vi "Write Config to File.vi"() -> ()   [LabVIEW 2014]
uses:
  General/Controls/System Parameters.ctl
  Hardware/Table Stage/Controls/Translation Stage Cluster.ctl
  General/Controls/Translation Stage Types.ctl
  <vilib>/Utility/config.llb/NI_LVConfig.lvlib
panel:
  in  "System Parameters":T1={"OCT"={"Focal Length"=0.0}, "Vibratome"={"Z Bottom"=0.0, "Pre Cut Dwell"=0.0, "Blade Frequency"=0.0, "Slice Speed"=0.0, "Post Cut Dwell"=0.0, "Ramp Time"=0.0, "Start X"=0.0, "Start Y"=0.0}, "Table Stages"={"X Stage"={"Position"=0.0, "Is.Enabled?"=FALSE, "Is.Connected?"=FALSE, "Device SN"="45876539", "AccelerationMaximum"=0.0, "VelocityMaximum"=0.0, "Acceleration"=0.0, "Velocity"=0.0, "waitTimeout (ms)"=0, "Model"=enum."None", "Is.Homed?"=FALSE}, "Y Stage"={"Position"=0.0, "Is.Enabled?"=FALSE, "Is.Connected?"=FALSE, "Device SN"="45876539", "AccelerationMaximum"=0.0, "VelocityMaximum"=0.0, "Acceleration"=0.0, "Velocity"=0.0, "waitTimeout (ms)"=0, "Model"=enum."None", "Is.Homed?"=FALSE}, "Z Stage"={"Position"=0.0, "Is.Enabled?"=FALSE, "Is.Connected?"=FALSE, "Device SN"="45876539", "AccelerationMaximum"=0.0, "VelocityMaximum"=0.0, "Acceleration"=0.0, "Velocity"=0.0, "waitTimeout (ms)"=0, "Model"=enum."None", "Is.Homed?"=FALSE}}}
  out "error out":errorcluster
  in  "error in (no error)":errorcluster
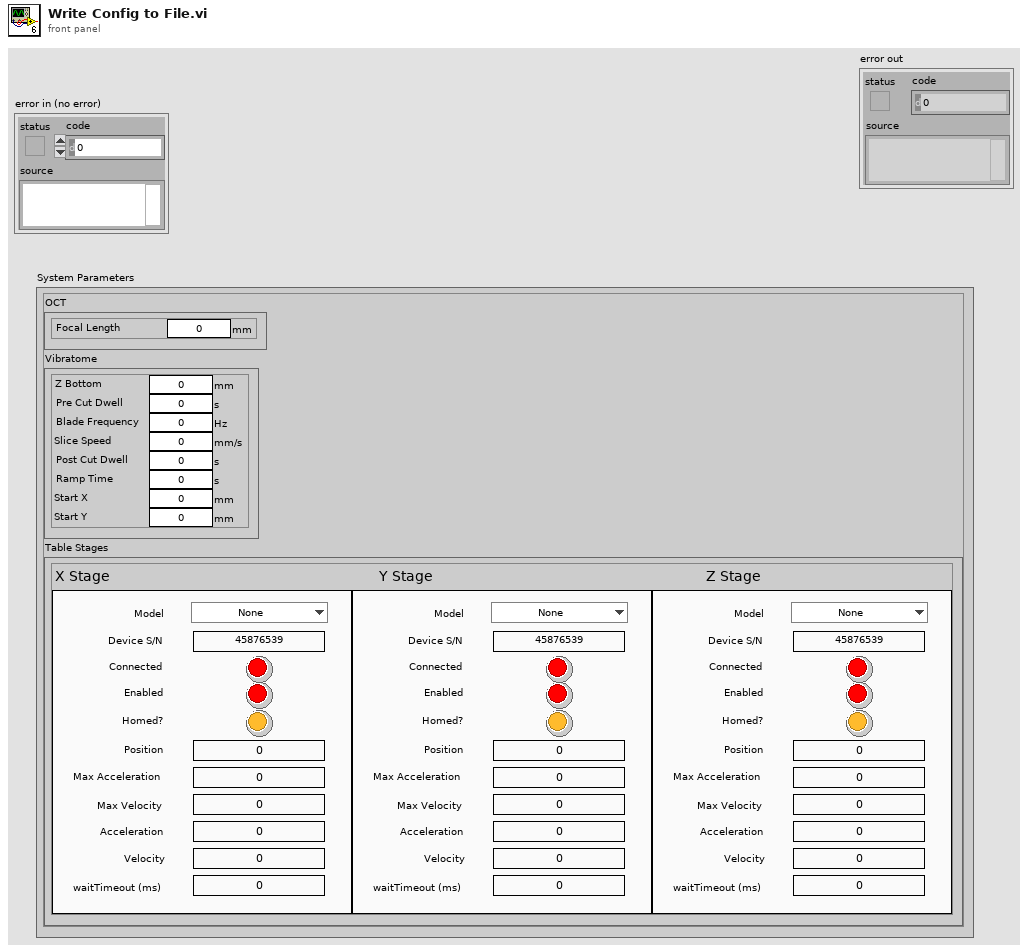
[diagram p1: front panel]
types:
  T1 = typedef "System Parameters.ctl" = cluster{"OCT":cluster{"Focal Length":dbl[unit]}, "Vibratome":cluster{"Z Bottom":dbl[unit], "Pre Cut Dwell":dbl[unit], "Blade Frequency":dbl[unit], "Slice Speed":dbl[unit], "Post Cut Dwell":dbl[unit], "Ramp Time":dbl[unit], "Start X":dbl[unit], "Start Y":dbl[unit]}, "Table Stages":cluster{"X Stage":T2, "Y Stage":T2, "Z Stage":T2}}
  T2 = typedef "Translation Stage Cluster.ctl" = cluster{"Position":dbl, "Is.Enabled?":bool, "Is.Connected?":bool, "Device SN":string, "AccelerationMaximum":dbl, "VelocityMaximum":dbl, "Acceleration":dbl, "Velocity":dbl, "waitTimeout (ms)":i32, "Model":T3, "Is.Homed?":bool}
  T3 = typedef "Translation Stage Types.ctl" = enum16{"None", "Thorlabs LTS", "Thorlabs MLJ"}
  T4 = typedef "NI_LVConfig.lvlib/Config Data RefNum.ctl" = refnum<k1>
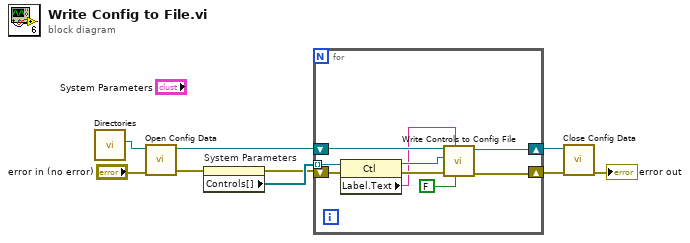
[diagram p0: block diagram]
diagram:
  n1 = call "Directories.vi"() -> ("Config.ini Path"=w7:path)  [unwired: 10 in, 1 out]
  n2 = call <vilib>:"Open Config Data.vi"("error in (no error)"="error in (no error)", "configuration file path"=w7) -> ("error out"=w1:errorcluster, "refnum"=w4:T4)  [unwired: 7 in, 1 out]
  n3 = property on="System Parameters" class="Clust (strict)"(error in=w1) -> (error out=w2:errorcluster, "Controls[]"=w6:refnum<vi>[])  [unwired: 1 in, 1 out]
  n4 = for {
    tunnel: w6 -> [w18] mode=indexing
    shift-right: [w14] -> w5
    shift-left: w2 -> [w17]
    shift-right: [w10] -> w3
    shift-left: w4 -> [w13]
    n5 = property class="Ctl"(reference=w18, error in=w17) -> (reference out=w12:refnum<vi>, error out=w15:errorcluster, "Label.Text"=w11:string)
    n6 = call "Write Controls to Config File.vi"("Child?"=FALSE, "section"=w11, "Error In"=w15, "Ctl Refnum"=w12, "refnum"=w13) -> ("Error Out"=w14:errorcluster, "refnum out"=w10:T4)  [unwired: 5 in]
  }
  n7 = call <vilib>:"Close Config Data.vi"("error in (no error)"=w5, "refnum"=w3) -> ("error out"=→"error out":errorcluster)  [unwired: 8 in, 1 out]
